vi "Create_Experiment_Data_Folder.vi"(0 "Data in":T1={"User Name"="", "Experiment Number"=0, "Start Time"=timestamp(0 s since 1904-01-01), "Data"=[], "Step Number"=1, "Step Instructions"="", "Diagnostics"={"Langmuir Probe"=FALSE, "Rogowski 1"=FALSE, "Rogowski 2"=FALSE, "Rogowski 3"=FALSE, "B-dot 1"=FALSE, "B-dot 2"=FALSE}, "Experiment Purpose"="", "Experiment State"=enum."Off", "Systems"={"Compressed Air"=FALSE, "T-20kV Power Switch"=FALSE, "T-Rectifier"=FALSE, "Engage Interlock"=FALSE, "Ventilator"=FALSE, "Magnetron"=FALSE, "H-20kV Power Switch"=FALSE, "H-Rectifier"=FALSE, "Main Water Pump"=FALSE, "WEGA Water Pump"=FALSE, "Gas Inlet Valves"=FALSE}, "Current Pressure"=0.0, "Fieldpoints"={"System Boolean Fieldpoints"={"Compressed Air"="", "T-20kV Power Switch"="", "T-Rectifier"="", "Engage Interlock"="", "Ventilator"="", "Magnetron"="", "H-20kV Power Switch"="", "H-Rectifier"="", "Main Water Pump"="", "WEGA Water Pump"="", "Gas Inlet Valves"=""}, "Step Fieldpoints"={"Exhaust Ventillator"="", "Compressed Air"="", "Water Pressure"="", "Interlock"=""}}, "Pressure History"={"Seconds into Experiment"=[], "Pressure Data"=[]}}, 1 "error in":errorcluster) -> (2 "Data out":T1={"User Name"="", "Experiment Number"=0, "Start Time"=timestamp(0 s since 1904-01-01), "Data"=[], "Step Number"=1, "Step Instructions"="", "Diagnostics"={"Langmuir Probe"=FALSE, "Rogowski 1"=FALSE, "Rogowski 2"=FALSE, "Rogowski 3"=FALSE, "B-dot 1"=FALSE, "B-dot 2"=FALSE}, "Experiment Purpose"="", "Experiment State"=enum."Off", "Systems"={"Compressed Air"=FALSE, "T-20kV Power Switch"=FALSE, "T-Rectifier"=FALSE, "Engage Interlock"=FALSE, "Ventilator"=FALSE, "Magnetron"=FALSE, "H-20kV Power Switch"=FALSE, "H-Rectifier"=FALSE, "Main Water Pump"=FALSE, "WEGA Water Pump"=FALSE, "Gas Inlet Valves"=FALSE}, "Current Pressure"=0.0, "Fieldpoints"={"System Boolean Fieldpoints"={"Compressed Air"="", "T-20kV Power Switch"="", "T-Rectifier"="", "Engage Interlock"="", "Ventilator"="", "Magnetron"="", "H-20kV Power Switch"="", "H-Rectifier"="", "Main Water Pump"="", "WEGA Water Pump"="", "Gas Inlet Valves"=""}, "Step Fieldpoints"={"Exhaust Ventillator"="", "Compressed Air"="", "Water Pressure"="", "Interlock"=""}}, "Pressure History"={"Seconds into Experiment"=[], "Pressure Data"=[]}}, 3 "Folder path":path, 4 "error out":errorcluster)   [LabVIEW 2015]
uses:
  Type_Defs/Data.ctl
  Type_Defs/Diagnostics.ctl
  Type_Defs/Systems.ctl
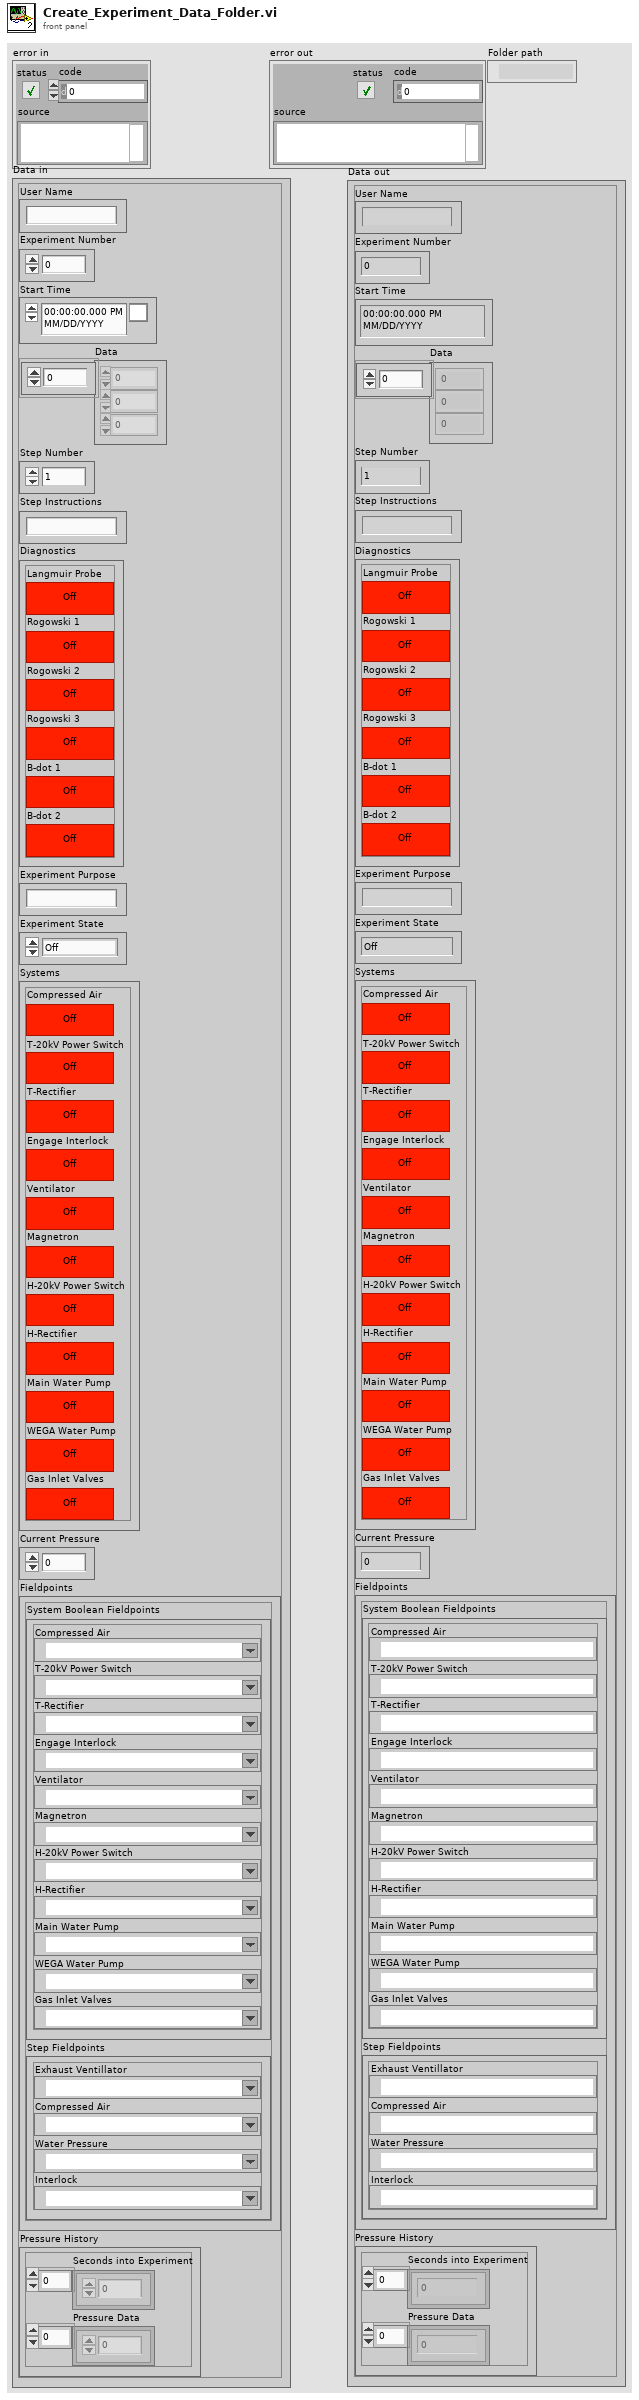
[diagram p1: front panel]
types:
  T1 = typedef "Data.ctl" = cluster{"User Name":string, "Experiment Number":i32, "Start Time":timestamp, "Data":dbl[], "Step Number":i32, "Step Instructions":string, "Diagnostics":T2, "Experiment Purpose":string, "Experiment State":enum16{"Off", "Setting Up", "Ready", "In Progress", "Shutting Down"}, "Systems":T3, "Current Pressure":dbl, "Fieldpoints":cluster{"System Boolean Fieldpoints":cluster{"Compressed Air":refnum<k21>, "T-20kV Power Switch":refnum<k21>, "T-Rectifier":refnum<k21>, "Engage Interlock":refnum<k21>, "Ventilator":refnum<k21>, "Magnetron":refnum<k21>, "H-20kV Power Switch":refnum<k21>, "H-Rectifier":refnum<k21>, "Main Water Pump":refnum<k21>, "WEGA Water Pump":refnum<k21>, "Gas Inlet Valves":refnum<k21>}, "Step Fieldpoints":cluster{"Exhaust Ventillator":refnum<k21>, "Compressed Air":refnum<k21>, "Water Pressure":refnum<k21>, "Interlock":refnum<k21>}}, "Pressure History":cluster{"Seconds into Experiment":i32[], "Pressure Data":dbl[]}}
  T2 = typedef "Diagnostics.ctl" = cluster{"Langmuir Probe":bool, "Rogowski 1":bool, "Rogowski 2":bool, "Rogowski 3":bool, "B-dot 1":bool, "B-dot 2":bool}
  T3 = typedef "Systems.ctl" = cluster{"Compressed Air":bool, "T-20kV Power Switch":bool, "T-Rectifier":bool, "Engage Interlock":bool, "Ventilator":bool, "Magnetron":bool, "H-20kV Power Switch":bool, "H-Rectifier":bool, "Main Water Pump":bool, "WEGA Water Pump":bool, "Gas Inlet Valves":bool}
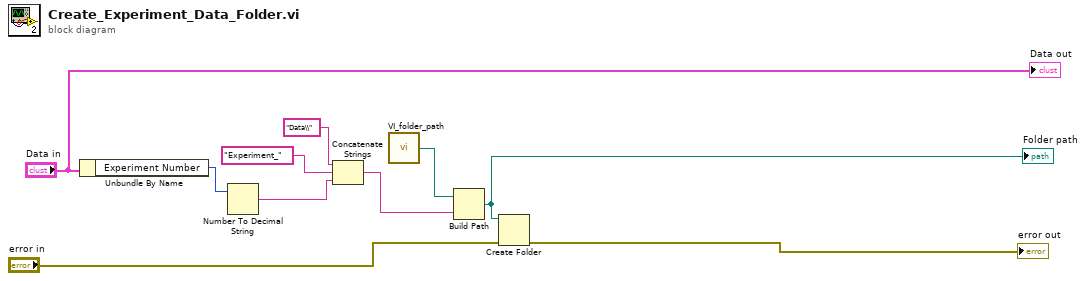
[diagram p0: block diagram]
diagram:
  n1 = Unbundle By Name("Data in") -> ("Experiment Number"=w8:i32)
  n2 = Number To Decimal String(number=w8) -> (decimal integer string=w7:string)  [unwired: 1 in]
  n3 = Concatenate Strings("Data\\" ("string"), "Experiment_" ("string"), w7) -> (w1:string)
  n4 = call "VI_folder_path.vi"() -> ("output path"=w5:path)
  n5 = Build Path(base path=w5, name or relative path=w1) -> (appended path=w4:path)
  "Folder path" <- w4
  n6 = Create Folder(path (use dialog)=w4, error in="error in") -> (error out=→"error out":errorcluster)  [unwired: 1 in, 2 out]
  "Data out" <- "Data in"
